vi "MU Get Interface Info.vi"(8 "error in (no error)":errorcluster, 10 "informationType":u32, 11 "handle":u64) -> (0 "error out (no error)":errorcluster, 2 "information":string, 3 "function return":u32)   [LabVIEW 2017, in "MU_3SL_interface.lvlib"]
uses:
  MU_3SL_interface.lvlib
  lib/MU_3SL_interface.dll
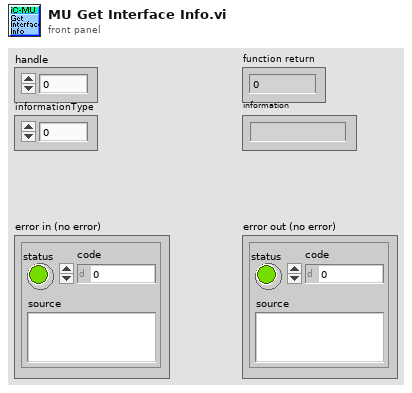
[diagram p1: front panel]
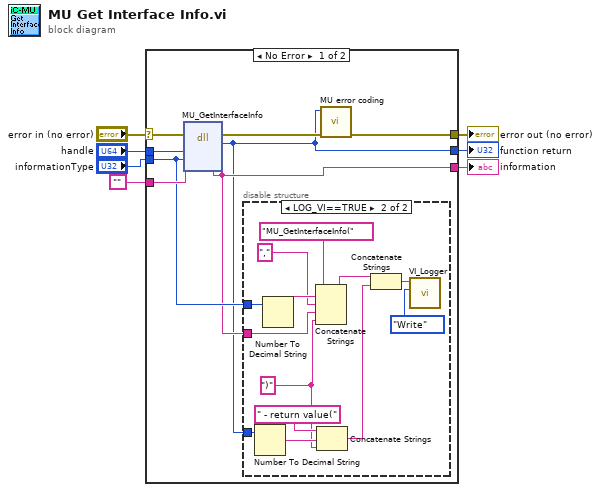
[diagram p0: block diagram]
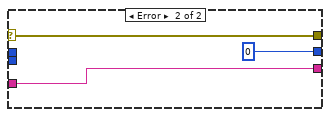
[diagram p3: hidden frame]
diagram:
  n1 = case shown="No Error" "error in (no error)" {
    selector: "error in (no error)" -> [w13 w31]
    tunnel: [w8 u32 0] -> w7
    tunnel: "handle" -> [w11 _]
    tunnel: "informationType" -> [w10 _]
    tunnel: [w9 w29] -> w4
    tunnel: [w14 w31] -> w3
    tunnel: "" -> [w12 w29]
    frame No Error {
      n2 = dll-call lib="C:/Users/bes/AppData/Roaming/work/mu_9so/icsubmodules/soft_mu_3sl_master/lv_interface/lib/MU_3SL_interface**.*" fn="MU_GetInterfaceInfo"(error in=w13, "handle"=w11, "informationType"=w10, "information"=w12) -> (error out=w15:errorcluster, "return type"=w8:u32, "information"=w9:string)  [unwired: 4 in, 1 out]
      n3 = disable-structure shown="LOG_VI==TRUE" {
        disable-tunnel: w8 -> [_ w26]
        disable-tunnel: w10 -> [_ w21]
        disable-tunnel: w9 -> [_ w19]
        frame condition #0 {
        }
        frame condition #1 (active) {
          w16 = ")" ("string")
          n4 = Number To Decimal String(number=w26) -> (decimal integer string=w25:string)  [unwired: 1 in]
          n5 = Number To Decimal String(number=w21) -> (decimal integer string=w20:string)  [unwired: 1 in]
          n6 = Concatenate Strings("MU_GetInterfaceInfo(" ("Info in"), w20, "," ("string"), w19, w16) -> (w24:string)
          n7 = Concatenate Strings(" - return value(" ("string"), w25, w16) -> (w23:string)
          n8 = Concatenate Strings(w24, w23) -> (w22:string)
          n9 = call "VI_Logger.vi"("Action (Read)"=enum16{"Write", "Read"}."Write", "Info in"=w22) -> ()  [unwired: 8 in, 2 out]
        }
      }
      n10 = call "MU error coding.vi"("error in (no error)"=w15, "function return in"=w8) -> ("error out"=w14:errorcluster)  [unwired: 9 in]
    }
    frame Error {
    }
  }
  "function return" <- w7
  "information" <- w4
  "error out (no error)" <- w3
